vi "FTW-ExtendedActorTemplate.vi"(0 "FTW Actor Instance Configuration":string="{\n  \"Identity\": \"ActorName\",\n  \"InboxAddress\": \"inproc://*\",\n  \"LoggerAddress\": \"\",\n  \"DebugEnableInboxLogging\": false,\n  \"DebugEnableJobLogging\": false,\n  \"LauncherAddress\": \"\",\n  \"Connections\": {\n    \"ConnectionOne\": \"inproc://connection-one\",\n    \"ConnectionTwo\": \"tcp://localhost/connection-two\"\n  },\n  \"Publishers\": {\n    \"PublisherOne\": \"inproc://publisher-one\",\n    \"PublisherTwo\": \"tcp://localhost/publisher-two\"\n  },\n  \"Subscriptions\": {\n    \"SubscriptionOne\": \"inproc://subscription-one\",\n    \"SubscriptionTwo\": \"tcp://localhost/subscription-two\"\n  }\n}", 11 "ErrorIn":errorcluster) -> (15 "Error":errorcluster)   [LabVIEW 2018]
uses:
  source/actor/Instance/FTW-ActorInstance.lvclass
  source/actor/Instance/FTW-ActorInstance.lvclass/FTW-ActorInstance.ctl
  source/actor/JobSequencer/FTW-SEQ-Current.vi
  source/actor/Message/Base/FTW-Message.lvclass
  source/actor/Message/Request/FTW-Message-IncomingRequest.lvclass
panel:
  # "Inputs"
  # "Outputs"
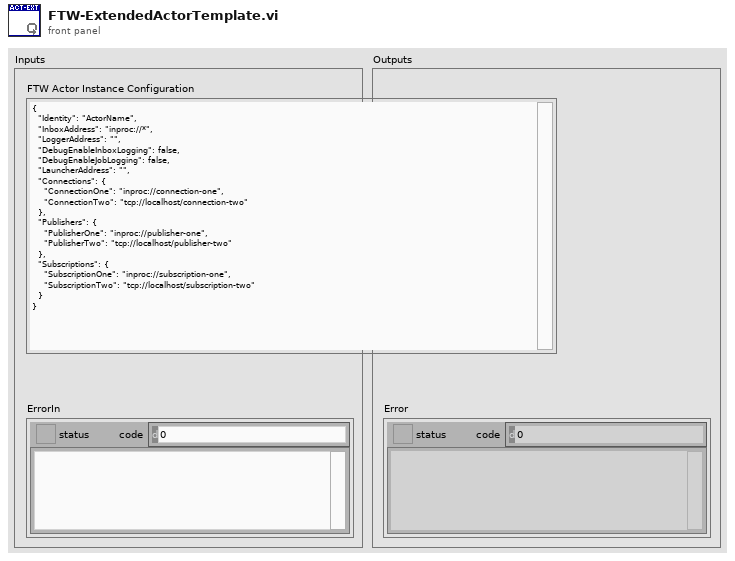
[diagram p1: front panel]
types:
  T1 = cluster{"Incoming Requests":refnum<event-registration>, "Local Messages":refnum<event-registration>, "Subscriber Registration":refnum<event-registration>}
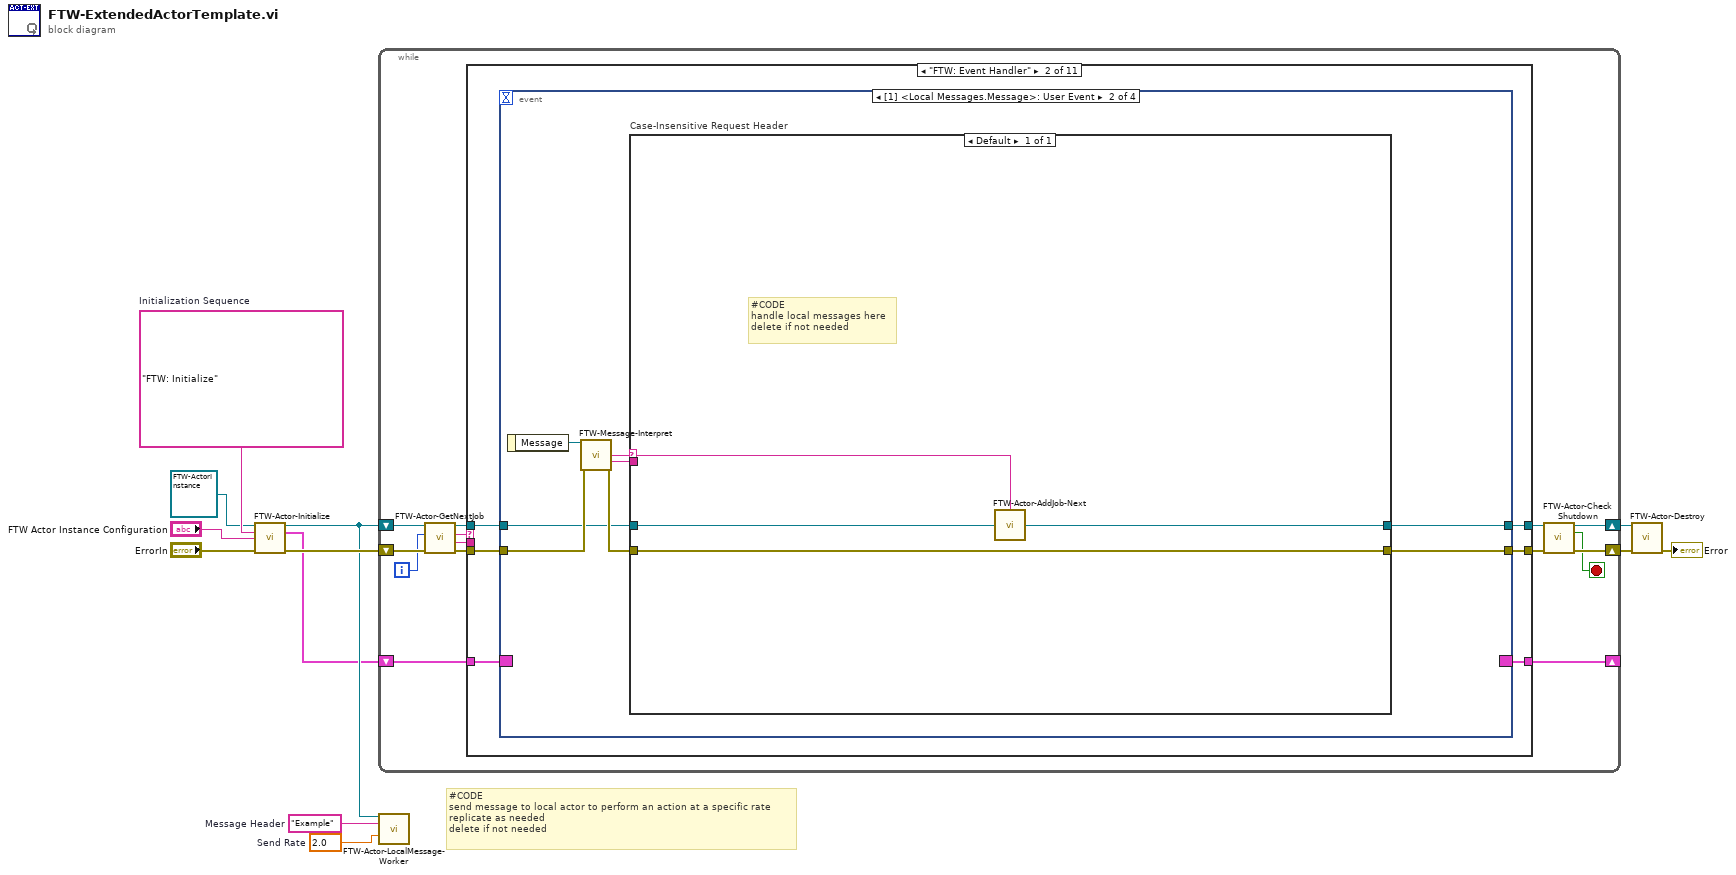
[diagram p0: block diagram]
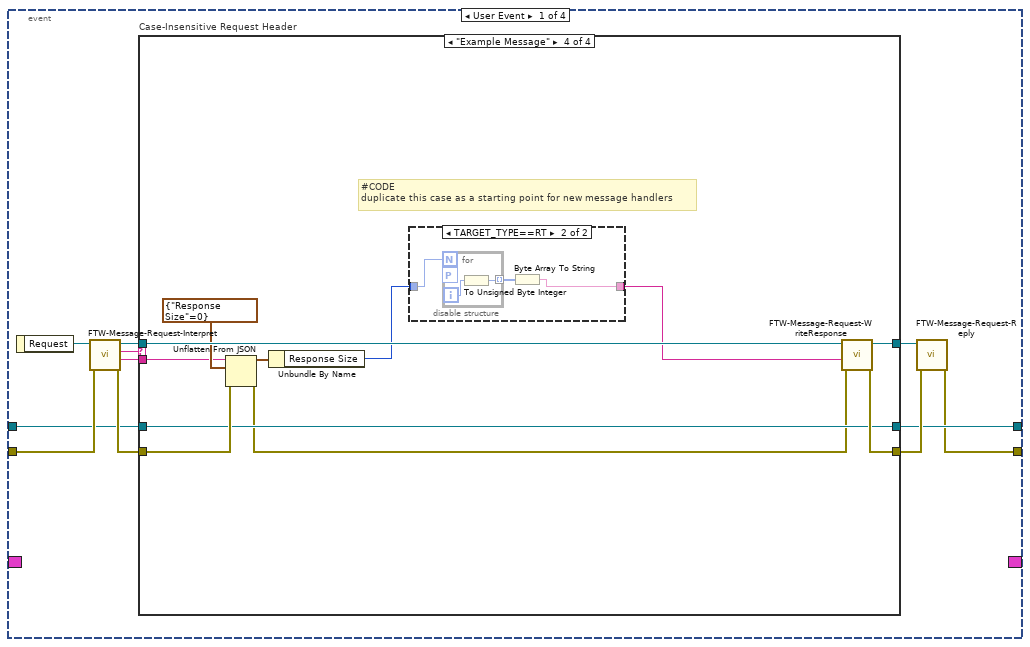
[diagram p3: hidden frame]
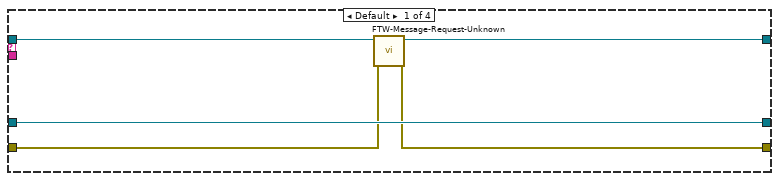
[diagram p4: hidden frame]
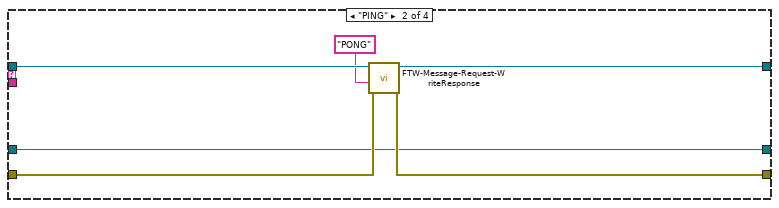
[diagram p5: hidden frame]
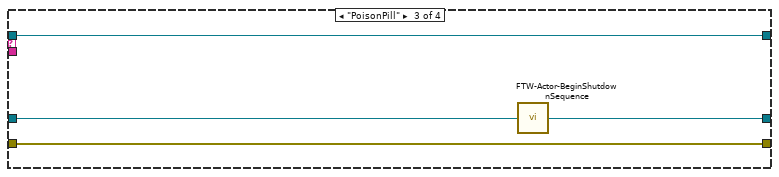
[diagram p6: hidden frame]
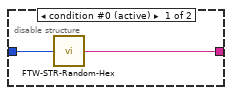
[diagram p7: hidden frame]
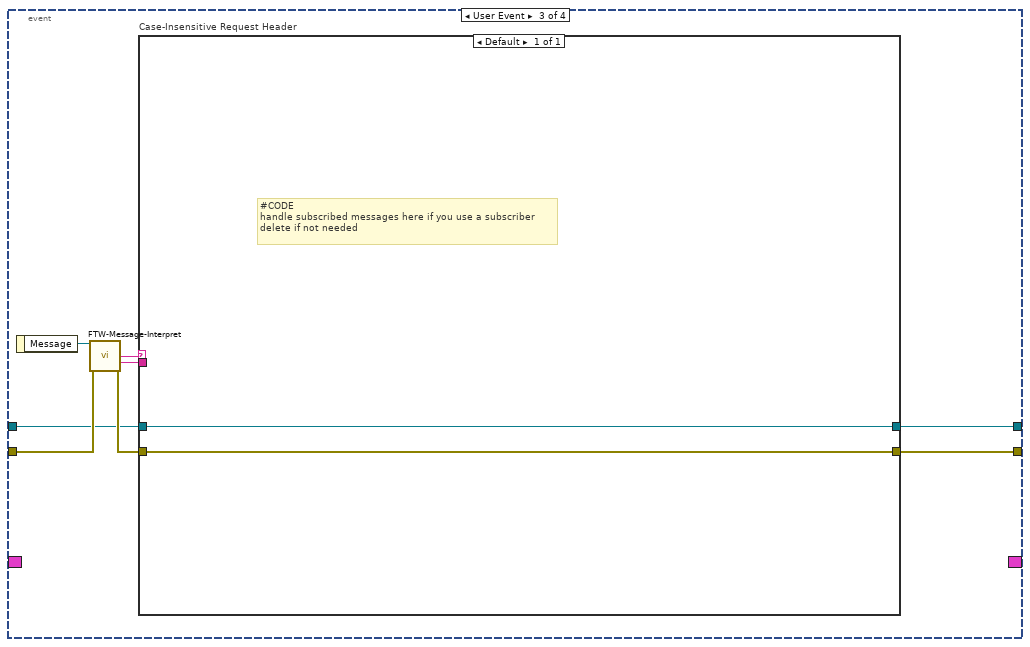
[diagram p8: hidden frame]
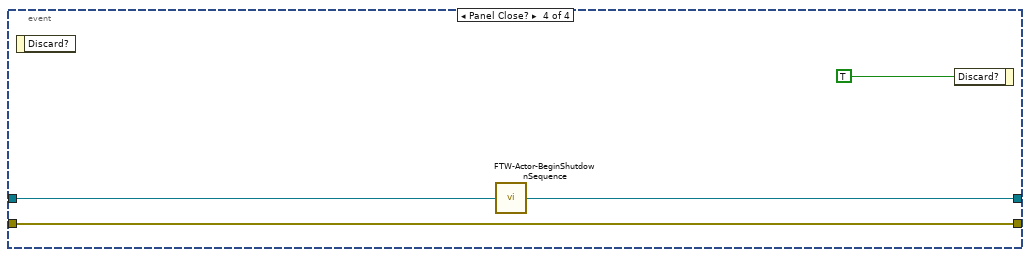
[diagram p9: hidden frame]
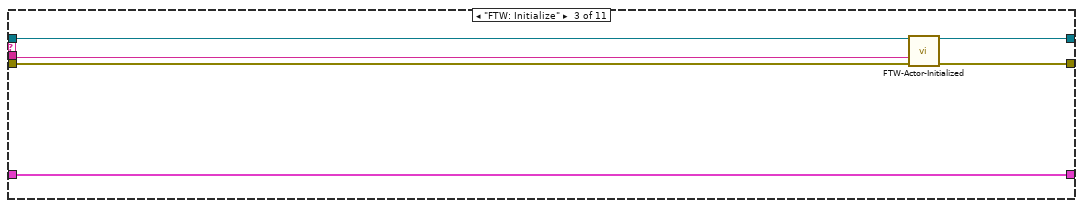
[diagram p10: hidden frame]
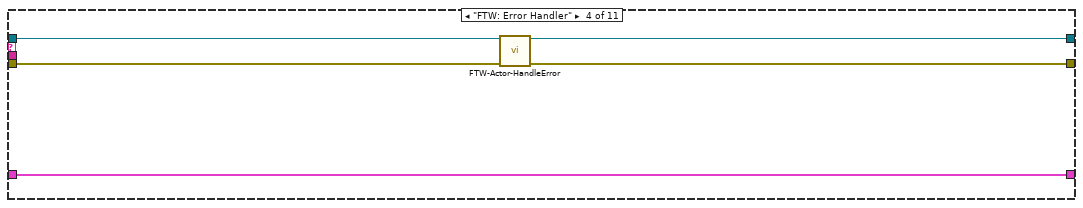
[diagram p11: hidden frame]
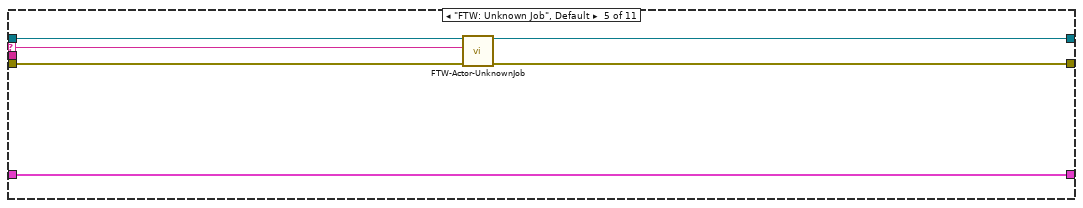
[diagram p12: hidden frame]
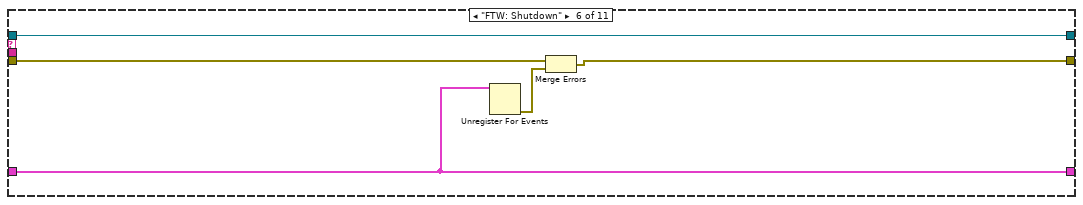
[diagram p13: hidden frame]
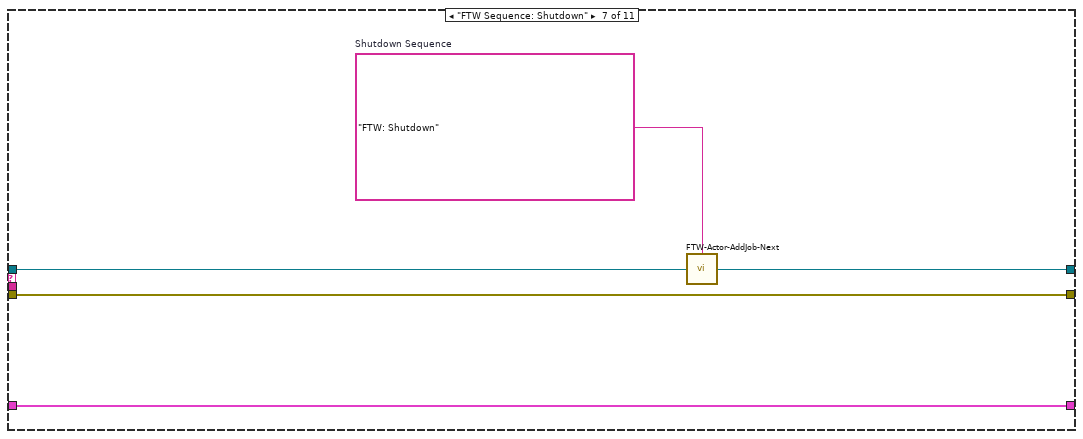
[diagram p14: hidden frame]
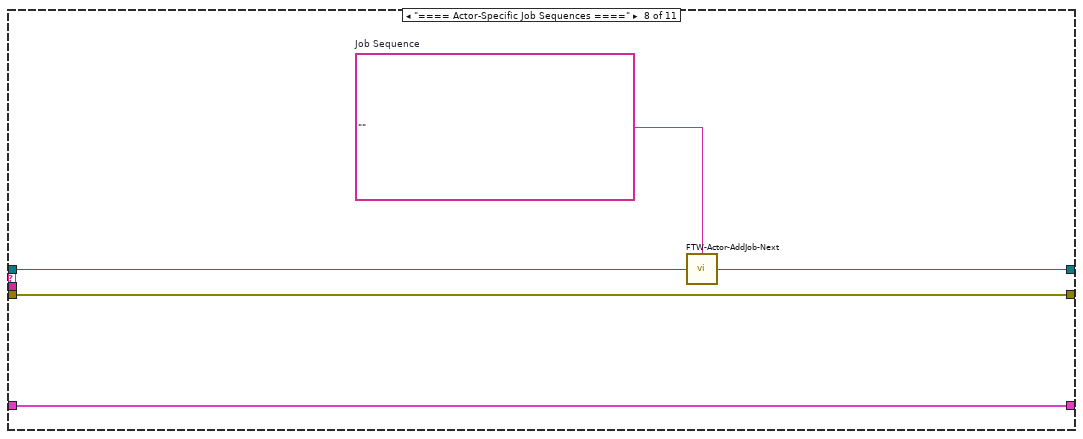
[diagram p15: hidden frame]
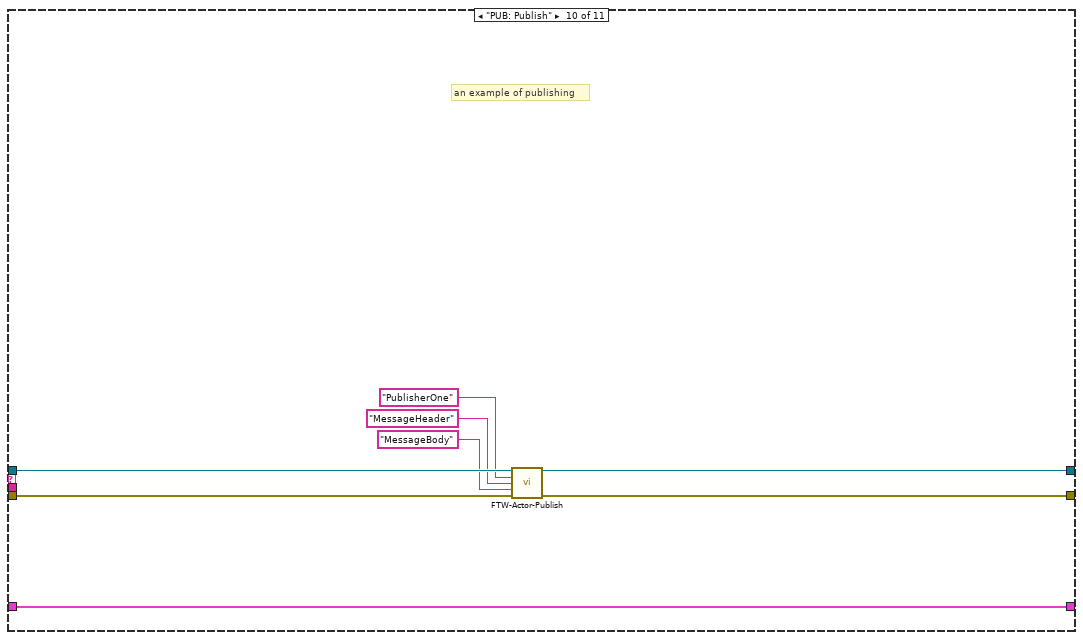
[diagram p17: hidden frame]
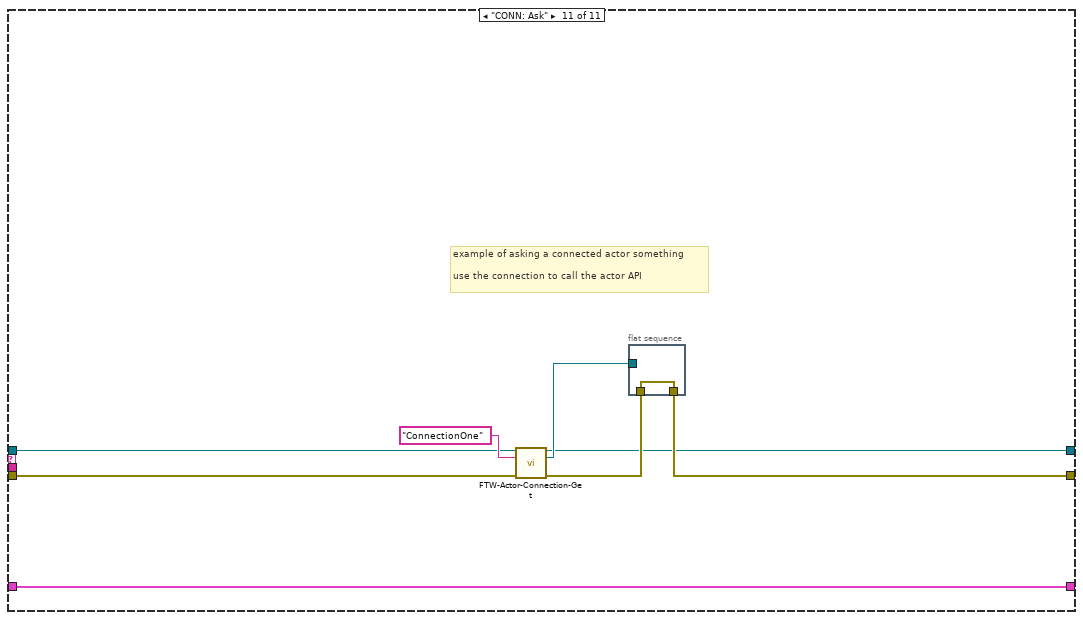
[diagram p18: hidden frame]
diagram:
  w3 = 2.0  # Send Rate
  w4 = "Example"  # Message Header
  w8 = "FTW: Initialize"  # Initialization Sequence
  # "#CODE\nsend message to local actor to perform an action at a specific rate\nreplicate as needed\ndelete if not needed"
  n1 = call-dynamic "FTW-Actor-Initialize.vi"("FTW Actor Instance Type"=refnum<class "FTW-ActorInstance.lvclass"> refnum, "Initialization Job Sequence"=w8, "Actor Instance Configuration"="FTW Actor Instance Configuration", "error in"="ErrorIn") -> ("FTW Actor Instance"=w5:refnum<class "FTW-ActorInstance.lvclass">, "Event Refnums"=w1:T1, "error out"=w9:errorcluster)  [unwired: 9 in]
  n2 = while {
    shift-right: [w16] -> w11
    shift-left: w9 -> [w23]
    shift-right: [w13] -> _
    shift-left: w1 -> [w26]
    shift-right: [w18] -> w12
    shift-left: w5 -> [w25]
    i -> [w14]
    stop <- w15 stop-if-true
    n3 = call "FTW-Actor-GetNextJob.vi"("error in"=w23, "Jobs Performed"=w14, "FTW Actor Instance"=w25) -> ("error out"=w22:errorcluster, "Job Data"=w20:string, "Job Name"=w21:string, "FTW Actor Instance out"=w24:refnum<class "FTW-ActorInstance.lvclass">)  [unwired: 5 in]
    n4 = case shown="\"FTW: Event Handler\"" w21 {
      selector: w21 -> [_ _ _ _ w117 _ _ _ _ _ _]
      tunnel: [w28 w35 w107 w112 w120 w126 w131 w136 w140 w144 w151] -> w17
      tunnel: w22 -> [w28 w34 w110 w114 w121 w127 w131 w136 w140 w145 w153]
      tunnel: w26 -> [w29 w30 w111 w116 w122 w123 w132 w137 w139 w148 w156]
      tunnel: [w29 w33 w111 w116 w122 w123 w132 w137 w139 w148 w156] -> w13
      tunnel: w20 -> [_ _ w106 _ _ _ _ _ _ _ _]
      tunnel: [w27 w32 w108 w113 w118 w124 w129 w134 w138 w146 w150] -> w19
      tunnel: w24 -> [w27 w31 w109 w115 w119 w124 w130 w135 w138 w147 w149]
      frame "==== Featherweight Framework Jobs ====" {
      }
      frame "FTW: Event Handler" {
        n5 = event shown="[1] <Local Messages.Message>: User Event" {
          selector: w30 -> [_ _ _ _]
          dyn-events: [_ _ _ _] -> w33
          timeout: _ -> [_ _ _ _]
          tunnel: [w38 w84 w96 w104] -> w35
          tunnel: w34 -> [w44 w85 w97 w104]
          tunnel: [w42 w83 w95 w102] -> w32
          tunnel: w31 -> [w41 w82 w94 w103]
          event User Event {
            n6 = event-data() -> ("Request"=w45:refnum<class "FTW-Message-IncomingRequest.lvclass">)  [unwired: 1 in]
            n7 = call "FTW-Message-Request-Interpret.vi"("error in"=w44, "FTW Incoming Request"=w45) -> ("error out"=w46:errorcluster, "Request Body"=w36:string, "Request Header"=w40:string, "FTW Incoming Request out"=w39:refnum<class "FTW-Message-IncomingRequest.lvclass">)  [unwired: 6 in]
            n8 = case "Case-Insensitive Request Header" shown="\"Example Message\"" w40 {
              tunnel: [w49 w55 w60 w71] -> w43
              tunnel: w46 -> [w50 w56 w60 w72]
              tunnel: [w51 w54 w61 w68] -> w42
              tunnel: w41 -> [w51 w54 w59 w68]
              tunnel: w39 -> [w48 w57 w58 w70]
              tunnel: [w47 w53 w58 w69] -> w37
              tunnel: w36 -> [_ _ _ w62]
              frame Default {
                n9 = call "FTW-Message-Request-Unknown.vi"("error in"=w50, "FTW Incoming Request"=w48) -> ("error out"=w49:errorcluster, "FTW Incoming Request Out"=w47:refnum<class "FTW-Message-IncomingRequest.lvclass">)  [unwired: 8 in]
              }
              frame "PING" {
                n10 = call "FTW-Message-Request-WriteResponse.vi"("error in"=w56, "Response Body"="PONG" ("Response Header"), "FTW Incoming Request"=w57) -> ("error out"=w55:errorcluster, "FTW Incoming Request out"=w53:refnum<class "FTW-Message-IncomingRequest.lvclass">)  [unwired: 7 in]
              }
              frame "PoisonPill" {
                n11 = call "FTW-Actor-BeginShutdownSequence.vi"("FTW Actor Instance"=w59) -> ("FTW Actor Instance out"=w61:refnum<class "FTW-ActorInstance.lvclass">)  [unwired: 3 in]
              }
              frame "Example Message" {
                # "#CODE\nduplicate this case as a starting point for new message handlers"
                n12 = Unflatten From JSON(JSON string=w62, type and defaults=cluster{"Response Size":i32} {"Response Size"=0}, error in (no error)=w72) -> (value=w65:cluster{"Response Size":i32}, error out=w67:errorcluster)  [unwired: 4 in]
                n13 = Unbundle By Name(w65) -> ("Response Size"=w64:i32)
                n14 = disable-structure shown="TARGET_TYPE==RT" {
                  disable-tunnel: w64 -> [w74 w77]
                  disable-tunnel: [w73 w75] -> w63
                  frame condition #0 (active) {
                    n15 = call "FTW-STR-Random-Hex.vi"("String Length"=w74) -> ("Random Hex String"=w73:string)  [unwired: 3 in]
                  }
                  frame condition #1 {
                    n16 = for {
                      N: w77 -> [_]
                      workers-P: _ -> [_]
                      tunnel: [w78] -> w76 mode=indexing
                      i -> [w79]
                      n17 = To Unsigned Byte Integer(number=w79) -> (unsigned 8bit integer=w78:u8)
                    }
                    n18 = Byte Array To String(unsigned byte array=w76) -> (string=w75:string)
                  }
                }
                n19 = call "FTW-Message-Request-WriteResponse.vi"("error in"=w67, "Response Body"=w63, "FTW Incoming Request"=w70) -> ("error out"=w71:errorcluster, "FTW Incoming Request out"=w69:refnum<class "FTW-Message-IncomingRequest.lvclass">)  [unwired: 7 in]
              }
            }
            n20 = call "FTW-Message-Request-Reply.vi"("FTW: Reply Error"=w43, "FTW Incoming Request"=w37) -> ("error out"=w38:errorcluster)  [unwired: 8 in, 1 out]
          }
          event User Event {
            n21 = event-data() -> ("Message"=w86:refnum<class "FTW-Message.lvclass">)  [unwired: 1 in]
            n22 = call-dynamic "FTW-Message-Interpret.vi"("FTW Message"=w86, "error in"=w85) -> ("Message Header"=w80:string, "Message Body"=w81:string, "error out"=w87:errorcluster)  [unwired: 9 in, 2 out]
            n23 = case "Case-Insensitive Request Header" shown="Default" w80 {
              selector: w80 -> [w88]
              tunnel: [w90] -> w84
              tunnel: w87 -> [w90]
              tunnel: [w89] -> w83
              tunnel: w82 -> [w91]
              tunnel: w81 -> [_]
              frame Default {
                # "#CODE\nhandle local messages here\ndelete if not needed"
                n24 = call "FTW-Actor-AddJob-Next.vi"("Add Next in Job Queue"=w88, "FTW Actor Instance"=w91) -> ("FTW Actor Instance out"=w89:refnum<class "FTW-ActorInstance.lvclass">)  [unwired: 2 in]
              }
            }
          }
          event User Event {
            n25 = event-data() -> ("Message"=w98:refnum<class "FTW-Message.lvclass">)  [unwired: 1 in]
            n26 = call-dynamic "FTW-Message-Interpret.vi"("FTW Message"=w98, "error in"=w97) -> ("Message Header"=w92:string, "Message Body"=w93:string, "error out"=w99:errorcluster)  [unwired: 9 in, 2 out]
            n27 = case "Case-Insensitive Request Header" shown="Default" w92 {
              tunnel: [w100] -> w96
              tunnel: w99 -> [w100]
              tunnel: [w101] -> w95
              tunnel: w94 -> [w101]
              tunnel: w93 -> [_]
              frame Default {
                # "#CODE\nhandle subscribed messages here if you use a subscriber\ndelete if not needed"
              }
            }
          }
          event Panel Close? {
            n28 = event-data() -> ()  [unwired: 1 in, 1 out]
            n29 = call "FTW-Actor-BeginShutdownSequence.vi"("FTW Actor Instance"=w103) -> ("FTW Actor Instance out"=w102:refnum<class "FTW-ActorInstance.lvclass">)  [unwired: 3 in]
            n30 = event-data("Discard?"=TRUE) -> ()  [unwired: 1 in, 1 out]
          }
        }
      }
      frame "FTW: Initialize" {
        n31 = call-dynamic "FTW-Actor-Initialized.vi"("FTW Actor Instance"=w109, "Positive Init?"=w106, "error in"=w110) -> ("FTW Actor Instance out"=w108:refnum<class "FTW-ActorInstance.lvclass">, "error out"=w107:errorcluster)  [unwired: 11 in]
      }
      frame "FTW: Error Handler" {
        n32 = call-dynamic "FTW-Actor-HandleError.vi"("FTW Actor Instance"=w115, "error in"=w114) -> ("FTW Actor Instance out"=w113:refnum<class "FTW-ActorInstance.lvclass">, "error out"=w112:errorcluster)  [unwired: 10 in, 2 out]
      }
      frame "FTW: Unknown Job", Default {
        n33 = call-dynamic "FTW-Actor-UnknownJob.vi"("FTW Actor Instance"=w119, "Unknown Job"=w117, "error in"=w121) -> ("FTW Actor Instance out"=w118:refnum<class "FTW-ActorInstance.lvclass">, "error out"=w120:errorcluster)  [unwired: 11 in]
      }
      frame "FTW: Shutdown" {
        n34 = Unregister For Events(event registration refnum=w123) -> (error out=w125:errorcluster)  [unwired: 1 in]
        n35 = Merge Errors(w127, w125) -> (w126:errorcluster)
      }
      frame "FTW Sequence: Shutdown" {
        w128 = "FTW: Shutdown"  # Shutdown Sequence
        n36 = call "FTW-Actor-AddJob-Next.vi"("Add Next in Job Queue"=w128, "FTW Actor Instance"=w130) -> ("FTW Actor Instance out"=w129:refnum<class "FTW-ActorInstance.lvclass">)  [unwired: 2 in]
      }
      frame "==== Actor-Specific Job Sequences ====" {
        w133 = ""  # Job Sequence
        n37 = call "FTW-Actor-AddJob-Next.vi"("Add Next in Job Queue"=w133, "FTW Actor Instance"=w135) -> ("FTW Actor Instance out"=w134:refnum<class "FTW-ActorInstance.lvclass">)  [unwired: 2 in]
      }
      frame "==== Actor-Specific Jobs ====" {
      }
      frame "PUB: Publish" {
        # "an example of publishing"
        n38 = call "FTW-Actor-Publish.vi"("FTW-ActorExtended In"=w147, "Publisher Name"="PublisherOne", "Message Header"="MessageHeader", "Message Body"="MessageBody", "error in"=w145) -> ("FTW-ActorExtended Out"=w146:refnum<class "FTW-ActorInstance.lvclass">, "error out"=w144:errorcluster)  [unwired: 9 in]
      }
      frame "CONN: Ask" {
        # "example of asking a connected actor something\n\nuse the connection to call the actor API"
        n39 = call "FTW-Actor-Connection-Get.vi"("FTW-ActorInstance In"=w149, "Connector Name"="ConnectionOne" ("Publisher Name"), "error in"=w153) -> ("FTW-ActorInstance Out"=w150:refnum<class "FTW-ActorInstance.lvclass">, "FTW Actor Connector"=w154:refnum<class "FTW-ActorConnector.lvclass">, "error out"=w152:errorcluster)  [unwired: 10 in]
        n40 = flat-sequence {
          tunnel: w154 -> [_]
          tunnel: w152 -> [w157]
          tunnel: [w157] -> w151
          frame #0 {
          }
        }
      }
    }
    n41 = call "FTW-Actor-CheckShutdown.vi"("FTW Actor Instance"=w19, "error in"=w17) -> ("FTW Actor Instance out"=w18:refnum<class "FTW-ActorInstance.lvclass">, "Shutdown?"=w15:bool, "error out"=w16:errorcluster)  [unwired: 11 in]
  }
  n42 = call "FTW-Actor-LocalMessage-Worker.vi"("FTW-ActorInstance In"=w5, "Message Header"=w4, "Send Rate"=w3) -> ()  [unwired: 13 in]
  n43 = call-dynamic "FTW-Actor-Destroy.vi"("FTW Actor Instance"=w12, "error in"=w11) -> ("error out"=→"Error":errorcluster)  [unwired: 13 in]
